vi "DIO Write Bank.vi"(8 "DIO.19:0.OUT":fxp<+,20,20> format="%020b", 9 "DO.DMA_CNTR":u16=5, 10 "DO.DMA_ENA":fxp<+,20,20> format="%b", 11 "DMA FIFO IN":refnum<k21>="DO") -> (0 "DO.DMA_IDL":bool, 2 "DATA OUT":fxp<+,20,20> format="%.0b")   [LabVIEW 2021]
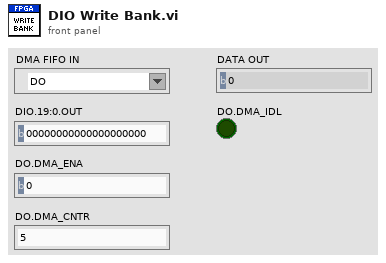
[diagram p1: front panel]
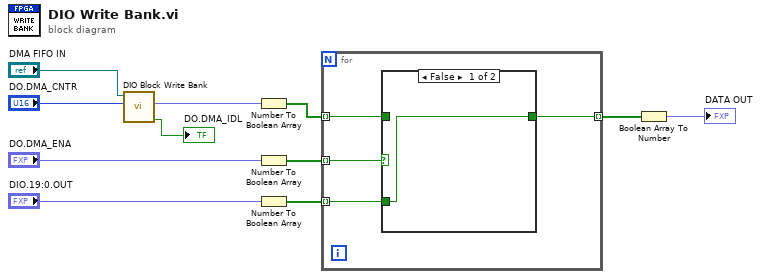
[diagram p0: block diagram]
diagram:
  n1 = call "DIO Block Write Bank.vi"("DO.DMA_CNTR"="DO.DMA_CNTR", "DMA FIFO IN"="DMA FIFO IN") -> ("DO.DMA_IDL"=→"DO.DMA_IDL":bool, "FIFO OUT"=w7:fxp<+,20,20>)  [unwired: 8 in]
  n2 = Number To Boolean Array(number=w7) -> (Boolean array=w3:bool[])
  n3 = Number To Boolean Array(number="DO.DMA_ENA") -> (Boolean array=w4:bool[])
  n4 = Number To Boolean Array(number="DIO.19:0.OUT") -> (Boolean array=w2:bool[])
  n5 = for {
    tunnel: w4 -> [w15] mode=indexing
    tunnel: w3 -> [w14] mode=indexing
    tunnel: w2 -> [w13] mode=indexing
    tunnel: [w12] -> w1 mode=indexing
    n6 = case shown="False" w15 {
      tunnel: w14 -> [_ w17]
      tunnel: w13 -> [w16 _]
      tunnel: [w16 w17] -> w12
      frame False {
      }
      frame True {
      }
    }
  }
  n7 = Boolean Array To Number(Boolean array=w1) -> (number=→"DATA OUT":fxp<+,20,20>)
